vi "Extracted CAD to temp folder.vi"(3 "Descriptions":T1=enum."CAD Outline", 5 "error in (no error)":errorcluster, 6 "Assembly":string, 7 "Extracted ODB":path, 9 "IPF temp folder":path, 11 "PCB Side":enum16{"Top", "Bottom"}(ring)) -> (14 "Temp file path":path, 19 "error out":errorcluster)   [LabVIEW 2013, in "Manipulate IPF.lvlib"]
uses:
  Manipulate IPF.lvlib
  Pack Data/type_def/file types.ctl
  <userlib>/_OpenG.lib/file/file.llb/Convert File Extension (String)__ogtk.vi
  Pack Data/Pack Files.lvlib
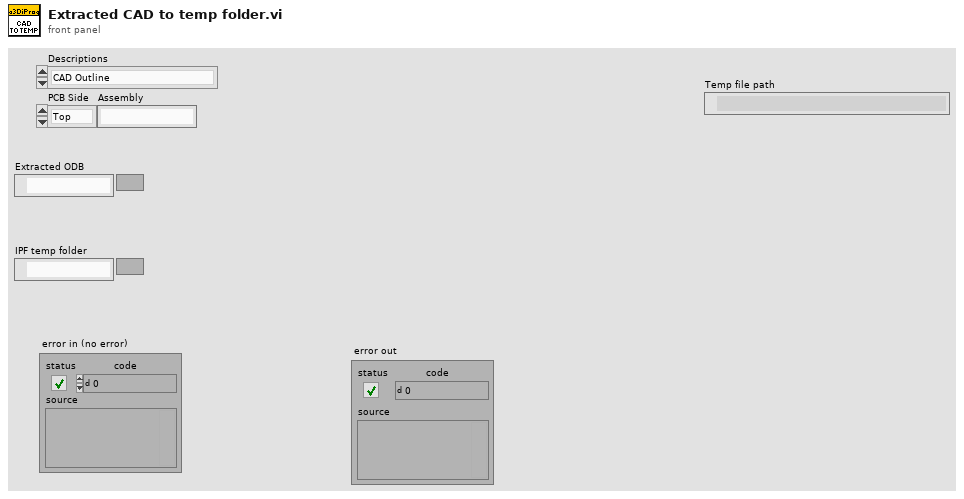
[diagram p1: front panel]
types:
  T1 = typedef "Pack Files.lvlib/file types.ctl" = enum16{"ODB", "TCF", "CAD Outline", "Config", "Inspection Prog", "a3Di-bin", "Results", "CAD Labels", "CAD Pads", "calScan_fid", "calScan_cal-tab", "PCB_SerialNumber", "CAD_Assembly", "Version", "Old Results", "CAD Picture", "Old TCF"}
  T2 = typedef "a3Di APG.lvlib/files.ctl" = cluster{"Programming Files":cluster{"PCB Design Identity":string, "ODB++ file":path, "Result temp  folder":path, "IPF temp folder":path}, "ODB file Converted?":bool, "Panel Params":T3, "PCB Outline File":path, "Initial Scan":bool, "PCBs on a carrier":bool, "Carrier Size":cluster{"X":dbl, "Y":dbl}, "IPF modified":bool, "PCB Side":enum16{"Top", "Bottom"}}
  T3 = typedef "Inspection.lvlib/Panel.lvclass/Config File data.ctl" = cluster{"Name":string, "Pos & Rot":T4, "PCBs List":cluster{"PCB Params":T5}[], "PCB BarCode Params":T6[], "Scan Type":bool}
  T4 = typedef "Inspection.lvlib/Pos and Rot.ctl" = cluster{"X":dbl, "Y":dbl, "Z":dbl, "rotation":dbl}
  T5 = typedef "Inspection.lvlib/PCB.lvclass/PCB Params.ctl" = cluster{"Name":string, "Pos & Rot":T4}
  T6 = typedef "Inspection.lvlib/Panel.lvclass/BarCode Params.ctl" = cluster{"ID":T7}
  T7 = typedef "Barcode Reader.lvlib/id.ctl" = u8
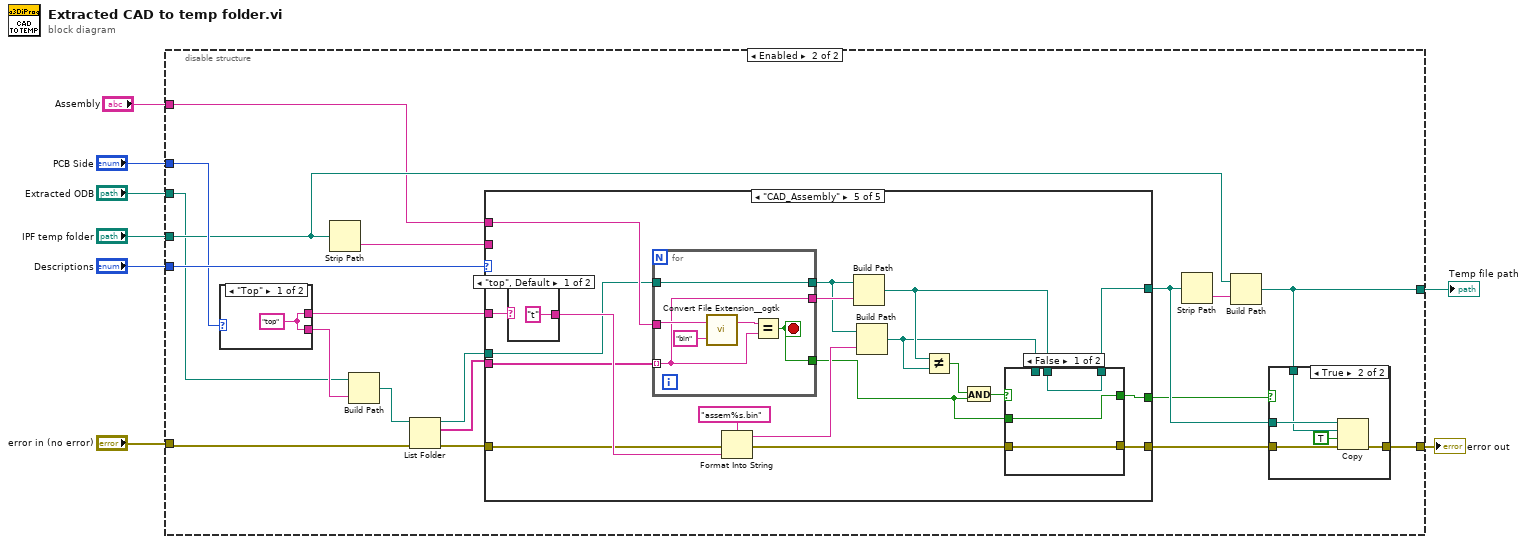
[diagram p0: block diagram]
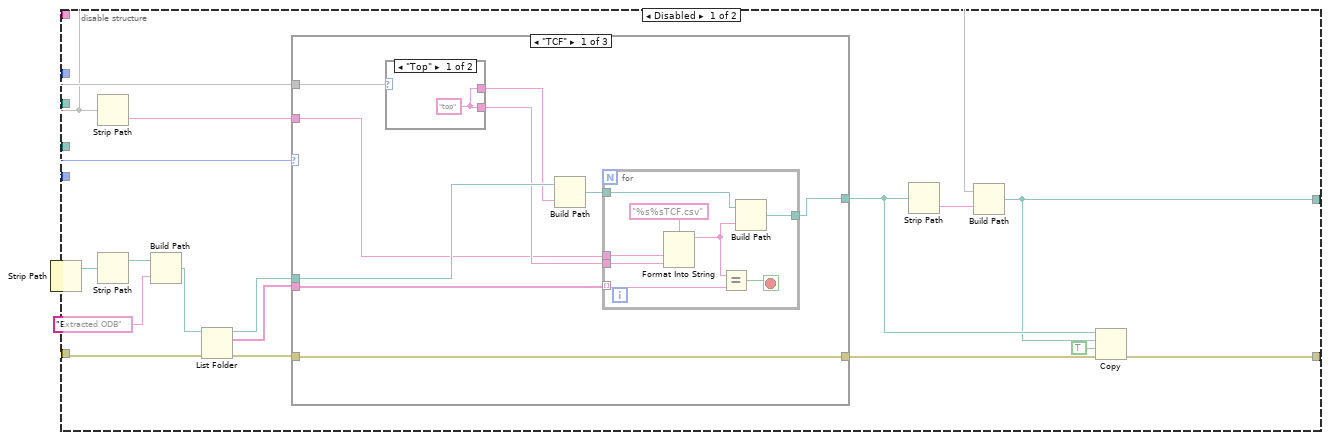
[diagram p2: hidden frame]
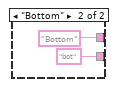
[diagram p3: hidden frame]
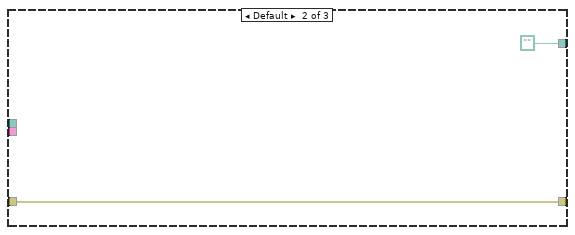
[diagram p4: hidden frame]
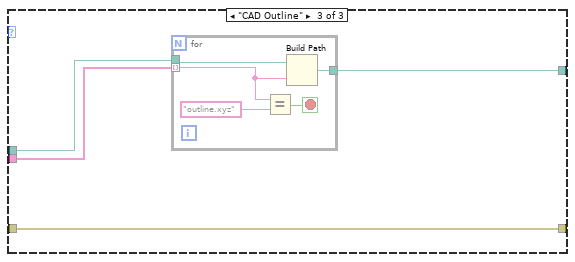
[diagram p5: hidden frame]
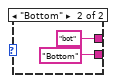
[diagram p7: hidden frame]
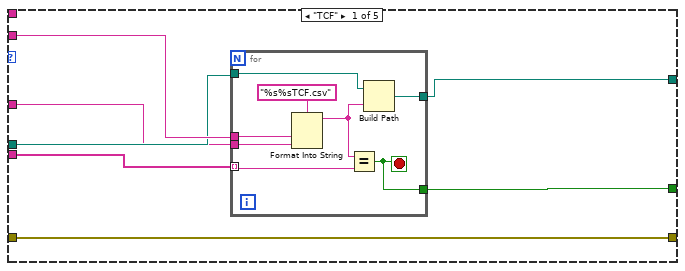
[diagram p8: hidden frame]
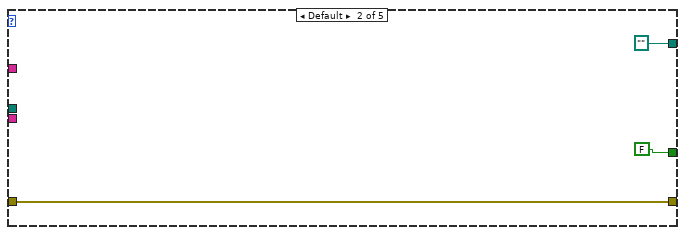
[diagram p9: hidden frame]
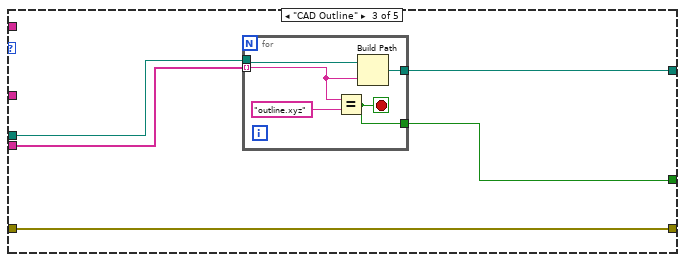
[diagram p10: hidden frame]
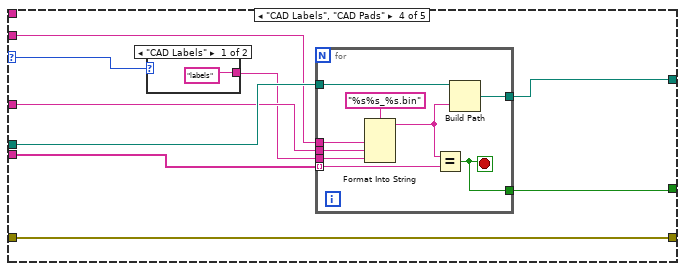
[diagram p11: hidden frame]
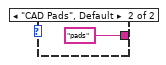
[diagram p12: hidden frame]
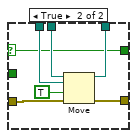
[diagram p13: hidden frame]
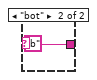
[diagram p14: hidden frame]
diagram:
  n1 = disable-structure shown="Enabled" {
    disable-tunnel: "error in (no error)" -> [w25 w71]
    disable-tunnel: [w15 w75] -> w7
    disable-tunnel: "Descriptions" -> [w10 w72]
    disable-tunnel: [w9 w65] -> w5
    disable-tunnel: "PCB Side" -> [_ w67]
    disable-tunnel: "Extracted ODB" -> [_ w62]
    disable-tunnel: "IPF temp folder" -> [_ w66]
    disable-tunnel: "Assembly" -> [_ w61]
    frame Disabled {
      n2 = Unbundle By Name() -> (w22:T2, "PCB Side"=w17, "Programming Files.IPF temp folder"=w16)
      n3 = List Folder(path=w16, error in=w25) -> (path out=w29:path, error out=w23:errorcluster)  [unwired: 2 in, 2 out]
      n4 = Strip Path(path=w29) -> (stripped path=w28:path)  [unwired: 1 out]
      n5 = Strip Path(path=w16) -> (name=w18:string)  [unwired: 1 out]
      n6 = Strip Path(path=w28) -> (stripped path=w27:path)  [unwired: 1 out]
      n7 = Build Path(base path=w27, name or relative path="Extracted ODB") -> (appended path=w24:path)
      n8 = List Folder(path=w24, error in=w23) -> (path out=w20:path, filenames=w19:string[], error out=w21:errorcluster)  [unwired: 2 in, 1 out]
      n9 = case shown="\"TCF\"" w10 {
        tunnel: [w35 path "" w55] -> w13
        tunnel: w17 -> [w36 _ _]
        tunnel: w19 -> [w37 _ w54]
        tunnel: w20 -> [w38 _ w53]
        tunnel: w21 -> [w30 w51 w52]
        tunnel: w18 -> [w31 _ _]
        tunnel: [w30 w51 w52] -> w11
        frame "TCF" {
          n10 = case shown="\"Top\"" w36 {
            tunnel: [w47 "bot"] -> w34
            tunnel: [w47 "Bottom"] -> w32
            frame "Top" {
              w47 = "top"
            }
            frame "Bottom" {
            }
          }
          n11 = Build Path(base path=w38, name or relative path=w32) -> (appended path=w33:path)
          n12 = for {
            tunnel: [w45] -> w35
            tunnel: w33 -> [w41]
            tunnel: w37 -> [w42] mode=indexing
            tunnel: w34 -> [w40]
            tunnel: w31 -> [w39]
            stop <- w46 stop-if-true
            n13 = Format Into String(format string="%s%sTCF.csv", w39, w40) -> (resulting string=w44:string)  [unwired: 2 in, 1 out]
            n14 = Equal?(x=w44, y=w42) -> (x = y?=w46:bool)
            n15 = Build Path(base path=w41, name or relative path=w44) -> (appended path=w45:path)
          }
        }
        frame Default {
        }
        frame "CAD Outline" {
          n16 = for {
            tunnel: w54 -> [w57] mode=indexing
            tunnel: w53 -> [w60]
            tunnel: [w59] -> w55
            stop <- w58 stop-if-true
            n17 = Equal?(x=w57, y="outline.xyz") -> (x = y?=w58:bool)
            n18 = Build Path(base path=w60, name or relative path=w57) -> (appended path=w59:path)
          }
        }
      }
      n19 = Strip Path(path=w13) -> (name=w12:string)  [unwired: 1 out]
      n20 = Build Path(base path=w16, name or relative path=w12) -> (appended path=w9:path)
      n21 = Copy(8:w11, 9:TRUE ("overwrite (F)"), 10:w9, 11:w13) -> (0:w15:errorcluster)  [unwired: 1 in, 2 out]
    }
    frame Enabled {
      n22 = case shown="\"Top\"" w67 {
        tunnel: [w86 "bot"] -> w69
        tunnel: [w86 "Bottom"] -> w70
        frame "Top" {
          w86 = "top"
        }
        frame "Bottom" {
        }
      }
      n23 = Strip Path(path=w66) -> (name=w76:string)  [unwired: 1 out]
      n24 = Build Path(base path=w62, name or relative path=w70) -> (appended path=w68:path)
      n25 = List Folder(path=w68, error in=w71) -> (path out=w78:path, filenames=w77:string[], error out=w79:errorcluster)  [unwired: 2 in, 1 out]
      n26 = case shown="\"CAD_Assembly\"" w72 {
        selector: w72 -> [_ _ _ w125 _]
        tunnel: [w94 path "" w111 w124 w155] -> w74
        tunnel: w77 -> [w95 _ w110 w123 w142]
        tunnel: w78 -> [w91 _ w109 w122 w143]
        tunnel: w79 -> [w92 w106 w108 w118 w144]
        tunnel: w76 -> [w93 _ _ w119 _]
        tunnel: [w92 w106 w108 w118 w153] -> w64
        tunnel: w69 -> [w90 _ _ w121 w146]
        tunnel: [w89 FALSE w107 w117 w147] -> w63
        tunnel: w61 -> [_ _ _ _ w145]
        frame "TCF" {
          n27 = for {
            tunnel: [w103] -> w94
            tunnel: w91 -> [w99]
            tunnel: w95 -> [w100] mode=indexing
            tunnel: w90 -> [w98]
            tunnel: w93 -> [w97]
            tunnel: [w96] -> w89
            stop <- w96 stop-if-true
            n28 = Format Into String(format string="%s%sTCF.csv", w97, w98) -> (resulting string=w102:string)  [unwired: 2 in, 1 out]
            n29 = Equal?(x=w102, y=w100) -> (x = y?=w96:bool)
            n30 = Build Path(base path=w99, name or relative path=w102) -> (appended path=w103:path)
          }
        }
        frame Default {
        }
        frame "CAD Outline" {
          n31 = for {
            tunnel: w110 -> [w114] mode=indexing
            tunnel: w109 -> [w116]
            tunnel: [w115] -> w111
            tunnel: [w112] -> w107
            stop <- w112 stop-if-true
            n32 = Equal?(x=w114, y="outline.xyz") -> (x = y?=w112:bool)
            n33 = Build Path(base path=w116, name or relative path=w114) -> (appended path=w115:path)
          }
        }
        frame "CAD Labels", "CAD Pads" {
          n34 = case shown="\"CAD Labels\"" w125 {
            tunnel: ["labels" "pads"] -> w120
            frame "CAD Labels" {
            }
            frame "CAD Pads", Default {
            }
          }
          n35 = for {
            tunnel: w123 -> [w134] mode=indexing
            tunnel: [w133] -> w124
            tunnel: w122 -> [w130]
            tunnel: w121 -> [w129]
            tunnel: w120 -> [w128]
            tunnel: w119 -> [w127]
            tunnel: [w126] -> w117
            stop <- w126 stop-if-true
            n36 = Format Into String(format string="%s%s_%s.bin", w127, w129, w128) -> (resulting string=w132:string)  [unwired: 2 in, 1 out]
            n37 = Equal?(x=w132, y=w134) -> (x = y?=w126:bool)
            n38 = Build Path(base path=w130, name or relative path=w132) -> (appended path=w133:path)
          }
        }
        frame "CAD_Assembly" {
          n39 = case shown="\"top\", Default" w146 {
            tunnel: ["t" "b"] -> w150
            frame "top", Default {
            }
            frame "bot" {
            }
          }
          n40 = for {
            tunnel: w142 -> [w169] mode=indexing
            tunnel: w145 -> [w172]
            tunnel: [w168] -> w137
            tunnel: w143 -> [w173]
            tunnel: [w173] -> w152
            tunnel: [w169] -> w154
            stop <- w168 stop-if-true
            n41 = call-poly <userlib>:"Convert File Extension__ogtk.vi"("new ending (none)"="bin", "file name"=w172) -> ("new filename"=w170:string)  [unwired: 1 out]
            n42 = Equal?(x=w170, y=w169) -> (x = y?=w168:bool)
          }
          n43 = Format Into String(format string="assem%s.bin", error in=w144, w150) -> (resulting string=w148:string, error out=w149:errorcluster)  [unwired: 1 in]
          n44 = Build Path(base path=w152, name or relative path=w154) -> (appended path=w141:path)
          n45 = Build Path(base path=w152, name or relative path=w148) -> (appended path=w140:path)
          n46 = Not Equal?(x=w141, y=w140) -> (x != y?=w138:bool)
          n47 = And(x=w138, y=w137) -> (x .and. y?=w139:bool)
          n48 = case shown="False" w139 {
            selector: w139 -> [_ w159]
            tunnel: [w157 w164] -> w155
            tunnel: w141 -> [w157 w163]
            tunnel: w140 -> [_ w162]
            tunnel: [w158 w161] -> w153
            tunnel: w149 -> [w158 w160]
            tunnel: [w156 w159] -> w147
            tunnel: w137 -> [w156 _]
            frame False {
            }
            frame True {
              n49 = Move(source path=w163, error in=w160, 9:TRUE ("overwrite (F)"), 10:w162) -> (error out=w161:errorcluster, 3:w164:path)  [unwired: 1 in, 1 out]
            }
          }
        }
      }
      n50 = Strip Path(path=w74) -> (name=w73:string)  [unwired: 1 out]
      n51 = Build Path(base path=w66, name or relative path=w73) -> (appended path=w65:path)
      n52 = case shown="True" w63 {
        tunnel: [w80 w85] -> w75
        tunnel: w74 -> [_ w83]
        tunnel: w65 -> [_ w82]
        tunnel: w64 -> [w80 w81]
        frame False {
        }
        frame True {
          n53 = Copy(8:w81, 9:TRUE ("overwrite (F)"), 10:w82, 11:w83) -> (0:w85:errorcluster)  [unwired: 1 in, 2 out]
        }
      }
    }
  }
  "error out" <- w7
  "Temp file path" <- w5
